vi "FPL-Config Measurement.vi"(0 "Chirp spec in":T3, 5 "Speaker":T2, 11 "error in (no error)":errorcluster) -> (4 "Cal Stimulus":T1={"Min Freq (Hz)"=50.0, "Max Freq (Hz)"=50000.0, "Freq Step (Hz)"=50.0, "Waveform"=enum."Chirp", "Attenuation (dB)"=20.0, "Sample Rate (Hz)"=100000.0}, 6 "Stimulus":dbl[](array[numeric]), 8 "Mic Avg":dbl[][](array[numeric]), 10 "dt (ms)":dbl, 13 "df (Hz)":dbl, 15 "error out":errorcluster)   [LabVIEW 2015]
uses:
  Thevenin VIs/LV Source/Typedefs/Thev-Stimulus.ctl
  Utility VIs/Type Defs/Speaker ring.ctl
  Type Defs/Cal Stimulus.ctl
  Misc VIs/Connection Manager/Type Defs/Input sources.ctl
  Misc VIs/Connection Manager/Type Defs/Output sources.ctl
  PXI DAQ VIs/DAQ Engine VIs/AO Gain and Multiplier VIs/PXI Multipliers to AO Gains (1D).vi
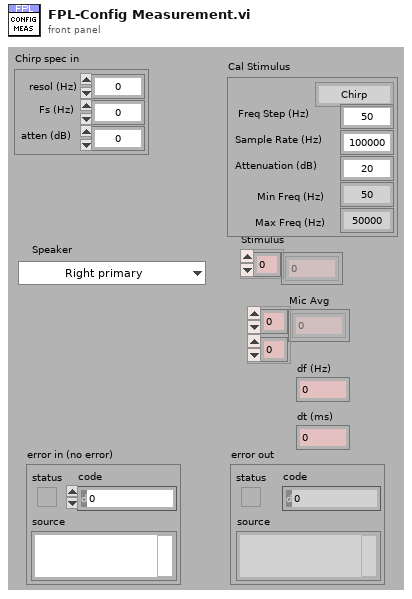
[diagram p1: front panel]
types:
  T1 = typedef "Cal Stimulus.ctl" = cluster{"Min Freq (Hz)":dbl, "Max Freq (Hz)":dbl, "Freq Step (Hz)":dbl, "Waveform":enum16{"Chirp", "Weighted"}, "Attenuation (dB)":dbl, "Sample Rate (Hz)":dbl}
  T2 = typedef "Speaker ring.ctl" = enum16{"Right primary", "Right secondary", "Left primary", "Left secondary"}
  T3 = typedef "Thev-Stimulus.ctl" = cluster{"resol (Hz)":dbl, "atten (dB)":dbl, "Fs (Hz)":dbl}
  T4 = typedef "Output sources.ctl" = u16
  T5 = typedef "Input sources.ctl" = u16
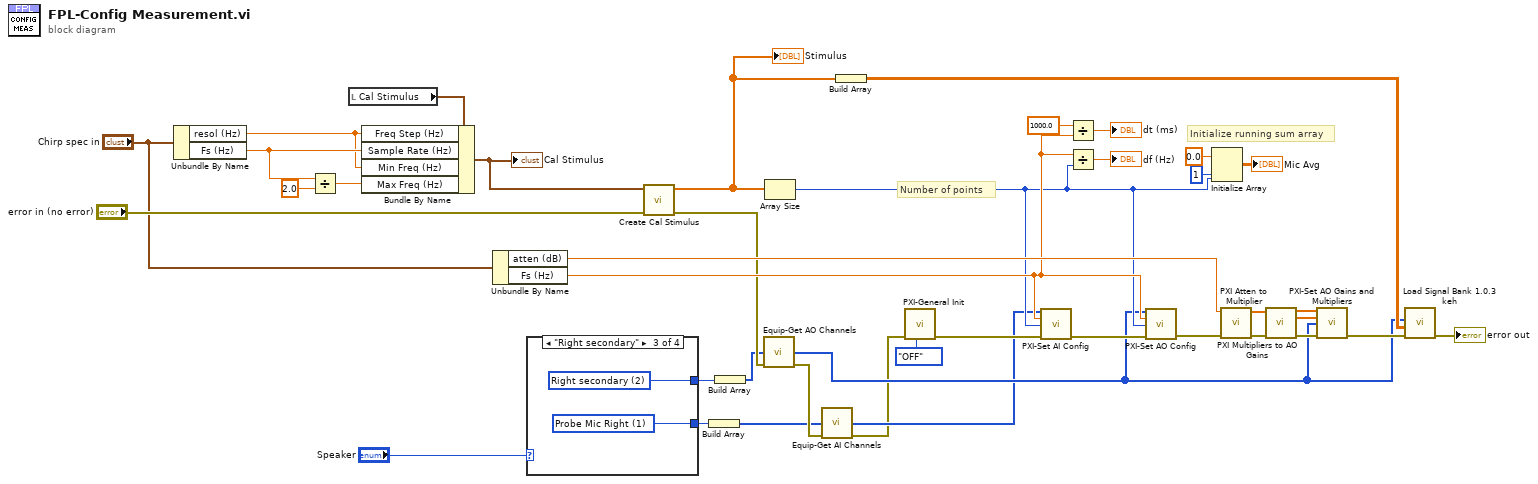
[diagram p0: block diagram]
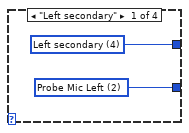
[diagram p2: hidden frame]
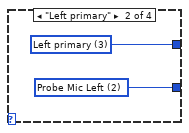
[diagram p3: hidden frame]
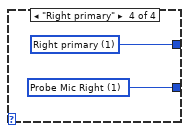
[diagram p4: hidden frame]
diagram:
  # "Number of points"
  # "Initialize running sum array"
  n1 = Unbundle By Name("Chirp spec in") -> ("resol (Hz)"=w1:dbl, "Fs (Hz)"=w2:dbl)
  n2 = Divide(x=w2, y=2.0) -> (x/y=w17:dbl)
  n3 = local read "Cal Stimulus"() -> (w4:T1)
  n4 = Bundle By Name(cluster=w4, "Freq Step (Hz)"=w1, "Sample Rate (Hz)"=w2, "Min Freq (Hz)"=w1, "Max Freq (Hz)"=w17) -> (w3:T1)
  "Cal Stimulus" <- w3
  n5 = Unbundle By Name("Chirp spec in") -> ("atten (dB)"=w37:dbl, "Fs (Hz)"=w22:dbl)
  n6 = case shown="\"Right secondary\"" "Speaker" {
    tunnel: [w42 w44 w46 w48] -> w7
    tunnel: [w41 w43 w45 w47] -> w6
    frame "Left secondary" {
      w42 = T4 4 items=["--unused--", "Right primary", "Right secondary", "Left primary", "Left secondary", "Shocks", "Startle", "Background"] ("Ring")
      w41 = T5 2 items=["--unused--", "Probe Mic Right", "Probe Mic Left", "Cal Mic", "ABR", "CAP Right", "CAP Left", "Startle piezo", "Temperature", "Heart rate"] ("Ring")
    }
    frame "Left primary" {
      w44 = T4 3 items=["--unused--", "Right primary", "Right secondary", "Left primary", "Left secondary", "Shocks", "Startle", "Background"] ("Ring")
      w43 = T5 2 items=["--unused--", "Probe Mic Right", "Probe Mic Left", "Cal Mic", "ABR", "CAP Right", "CAP Left", "Startle piezo", "Temperature", "Heart rate"] ("Ring")
    }
    frame "Right secondary" {
      w46 = T4 2 items=["--unused--", "Right primary", "Right secondary", "Left primary", "Left secondary", "Shocks", "Startle", "Background"] ("Ring")
      w45 = T5 1 items=["--unused--", "Probe Mic Right", "Probe Mic Left", "Cal Mic", "ABR", "CAP Right", "CAP Left", "Startle piezo", "Temperature", "Heart rate"] ("Ring")
    }
    frame "Right primary" {
      w48 = T4 1 items=["--unused--", "Right primary", "Right secondary", "Left primary", "Left secondary", "Shocks", "Startle", "Background"] ("Ring")
      w47 = T5 1 items=["--unused--", "Probe Mic Right", "Probe Mic Left", "Cal Mic", "ABR", "CAP Right", "CAP Left", "Startle piezo", "Temperature", "Heart rate"] ("Ring")
    }
  }
  n7 = call "Create Cal Stimulus.vi"("error in (no error)"="error in (no error)", "Cal Stimulus"=w3) -> ("error out"=w13:errorcluster, "Stimulus"=w40:dbl[])  [unwired: 7 in, 1 out]
  "Stimulus" <- w40
  n8 = Build Array(w6) -> (w9:T5[])
  n9 = Build Array(w7) -> (w8:T4[])
  n10 = call "Equip-Get AO Channels.vi"("Outputs"=w8, "error in (no error)"=w13) -> ("AO Channels"=w15:i32[], "error out"=w10:errorcluster)  [unwired: 12 in]
  n11 = Array Size(array=w40) -> (size(s)=w21:i32)
  n12 = call "Equip-Get AI Channels.vi"("Inputs"=w9, "error in (no error)"=w10) -> ("AI Channels"=w14:i32[], "error out"=w12:errorcluster)  [unwired: 12 in]
  n13 = Build Array(w40) -> (w19:dbl[][])
  n14 = call "PXI-General Init.vi"("Double Buffer Mode"=enum32{"OFF", "ENABLED", "FORCED"}."OFF", "error in (no error)"=w12) -> ("error out"=w25:errorcluster)  [unwired: 9 in]
  n15 = call "PXI-Set AI Config.vi"("AI Channels"=w14, "Sampling Rate (Hz)"=w22, "Buffer Size"=w21, "error in (no error)"=w25) -> ("error out"=w23:errorcluster)  [unwired: 11 in]
  n16 = Divide(x=1000.0, y=w22) -> (x/y=→"dt (ms)":dbl)
  n17 = Divide(x=w22, y=w21) -> (x/y=→"df (Hz)":dbl)
  n18 = call "PXI-Set AO Config.vi"("AO Channels"=w15, "Sampling Rate (Hz)"=w22, "Buffer Size"=w21, "error in (no error)"=w23) -> ("error out"=w24:errorcluster)  [unwired: 11 in]
  n19 = Initialize Array(0.0 ("element"), 1 ("dimension size"), w21) -> (→"Mic Avg":dbl[][])
  n20 = call "PXI Atten to Multiplier.vi"("error in (no error)"=w24, "Attenuation"=w37) -> ("error out"=w39:errorcluster, "Multiplier setting"=w38:dbl[])  [unwired: 8 in]
  n21 = call-poly "PXI Multipliers to AO Gains.vi"("Multipliers in"=w38, "error in (no error)"=w39) -> ("Multipliers out"=w27:dbl[], "Gains"=w26:dbl[], "error out"=w28:errorcluster)  [unwired: 11 in]
  n22 = call "PXI-Set AO Gains and Multipliers.vi"("Multipliers"=w27, "Gains"=w26, "AO Channels"=w15, "error in (no error)"=w28) -> ("error out"=w20:errorcluster)  [unwired: 11 in]
  n23 = call "Load Signal Bank 1.0.3 keh.vi"("error in (no error)"=w20, "Input array"=w19, "Active AO Array"=w15) -> ("error out"=→"error out":errorcluster)  [unwired: 6 in, 2 out]
